vi "Lidar V4.0 RT Main.vi"() -> ()   [LabVIEW 2013]
uses:
  <vilib>/Platform/TimedLoop/XDataNode/timing_clust.ctl
  <vilib>/Platform/TimedLoop/XDataNode/nitl_modes.ctl
  <vilib>/Platform/TimedLoop/XDataNode/wakeup.ctl
  <vilib>/FPGAPlugInAG/PXIe-7962R/niLvFpga_Open_PXIe-7962R.vi
  <vilib>/rvi/interface/common/dynamic/niFpgaDynamicAddResources.vi
  <vilib>/FPGAPlugInAG/Dynamic/niLvFpga_Abort_Dynamic.vi
  <vilib>/FPGAPlugInAG/Dynamic/niLvFpga_Reset_Dynamic.vi
  <vilib>/rvi/interface/common/niFpgaWaitOnOcc.vi
  <vilib>/Utility/error.llb/Error Cluster From Error Code.vi
  <vilib>/FPGAPlugInAG/Dynamic/niLvFpga_Run_Dynamic.vi
  <vilib>/rvi/errors/niLvFpgaAdjustHostInterfaceError.vi
  <vilib>/Utility/file.llb/Read From Spreadsheet File (I64).vi
  <vilib>/FPGAPlugInAG/Dynamic/niLvFpga_Close_Dynamic.vi
  <vilib>/rvi/interface/nirviOpenFPGA/nirviOpenFPGA.xnode
  FPGA Bitfiles/GMLIDARV4_FPGATarget4_LIDARV4FPGAMain_YvCqZtg0Yfs.lvbitx
  FPGA/LIDAR V4 FPGA Main.vi
  <vilib>/rvi/interface/nirviMethod/nirviMethod.xnode
  <vilib>/Platform/TimedLoop/XDataNode/XDataNode.xnode
  <vilib>/rvi/interface/nirviReadWriteControl/nirviReadWriteControl.xnode
  <vilib>/rvi/interface/nirviCloseFPGA/nirviCloseFPGA.xnode
  <vilib>/rvi/errors/niLvFpgaMergeErrorWithErrorCode.vi
  NiFpgaLv.dll
  <vilib>/rvi/interface/Simulation/niFpgaSimulationCallBeginRW.vi
  <vilib>/Platform/TimedLoop/XDataNode/XDNodeRunTimeDep.lvlib
  <vilib>/FPGAPlugInAG/Dynamic/niLvFpga_StopFifo_Dynamic.vi
  <vilib>/FPGAPlugInAG/Dynamic/niLvFpga_ConfigureFifo_Dynamic.vi
  <vilib>/FPGAPlugInAG/Dynamic/niLvFpga_AcquireReadRegionFifo_Dynamic.vi
panel:
  in  "Read Scan File":bool
  out "Address":i16[](array[numeric])
  out "Array":i32[](array[numeric])
  out "x .and. y?":i32[][](graph)
  out "data":i16[](graph)
  in  "Read From Pattern File":bool
  out "Timeouts":u16
  out "Elements In Region":u32
  in  "Led Pattern":u8[](array[numeric])=[0, 44, 88, 132, 176, 220, 8, 52, 96, 140, 184, 228, 16, 60, 104, 148, 192, 236, 24, 68, 112, 156, 200, 244, 32, 76, 120, 164, 208, 252, 40, 84, 128, 172, 216, 4, 48, 92, 136, 180, 224, 12, 56, 100, 144, 188, 232, 20, 64, 108, 152, 196, 240, 28, 72, 116, 160, 204, 248, 36, 80, 124, 168, 212, 0, 44, 88, 132, 176, 220, 8, 52, 96, 140, 184, 228, 16, 60, 104, 148, 192, 236, 24, 68, 112, 156, 200, 244, 32, 76, 120, 164, 208, 252, 40, 84, 128, 172, 216, 4]
  in  "Fill Led Pattern":bool
  in  "# of Frames":u32=1 caption="# of Frames:"
  in  "Frames2File":bool
  in  "Fill VGA":bool
  in  "VGA data":i16[](array[numeric])=[0, 300, 600, 900, 1200, 1500, 1800, 2100, 2400, 2700, 3000, 3300, 3600, 3900, 4200, 4500, 4800, 5100, 5400, 5700, 6000, 6300, 6600, 6900, 7200, 7500, 7800, 8100, 8400, 8700, 9000, 9300, 9600, 9900, 10200, 10500, 10800, 11100, 11400, 11700, 12000, 12300, 12600, 12900, 13200, 13500, 13800, 14100, 14400, 14700, 15000, 15300, 15600, 15900, 16200, 16500, 16800, 17100, 17400, 17700, 18000, 18300, 18600, 18900, 19200, 19500, 19800, 20100, 20400, 20700, 21000, 21300, 21600, 21900, 22200, 22500, 22800, 23100, 23400, 23700, 24000, 24300, 24600, 24900, 25200, 25500, 25800, 26100, 26400, 26700, 27000, 27300, 27600, 27900, 28200, 28500, 28800, 29100, 29400, 29700]
  in  "PulsePerLed":i16=200 caption="Pulses Per Led"
  in  "ScanMode":bool
  in  "FrameStartDisable":bool=TRUE
  out "# of Frames 2":u32
  in  "Frames Stream":bool
  in  "Frames Period":i64=100
  out "Actual DMA Depth":u32=4000768
  out "Raw Data Timeouts":u16
  in  "StreamToRawFile":bool=TRUE
  out "Elements":i32=8192
  out "DiskWritesCounter":dbl=6240.0
  out "error out":errorcluster
  in  "Write To File":bool
  in  "Output file path":path=path "C:/Users/LIDAR/Desktop/Scans/Debug1.dat"
  out "Elements Remaining":u32
  in  "MaxStartSample":u8
  in  "ActiveLedIndex":u16=144
  in  "LedScanDebEn":bool
  in  "LaserPower 1":bool=TRUE
  in  "LaserPower 0":bool=TRUE
  in  "SampPerPattern":u32=4
  in  "stop":bool=TRUE
  # "Auto Actions"
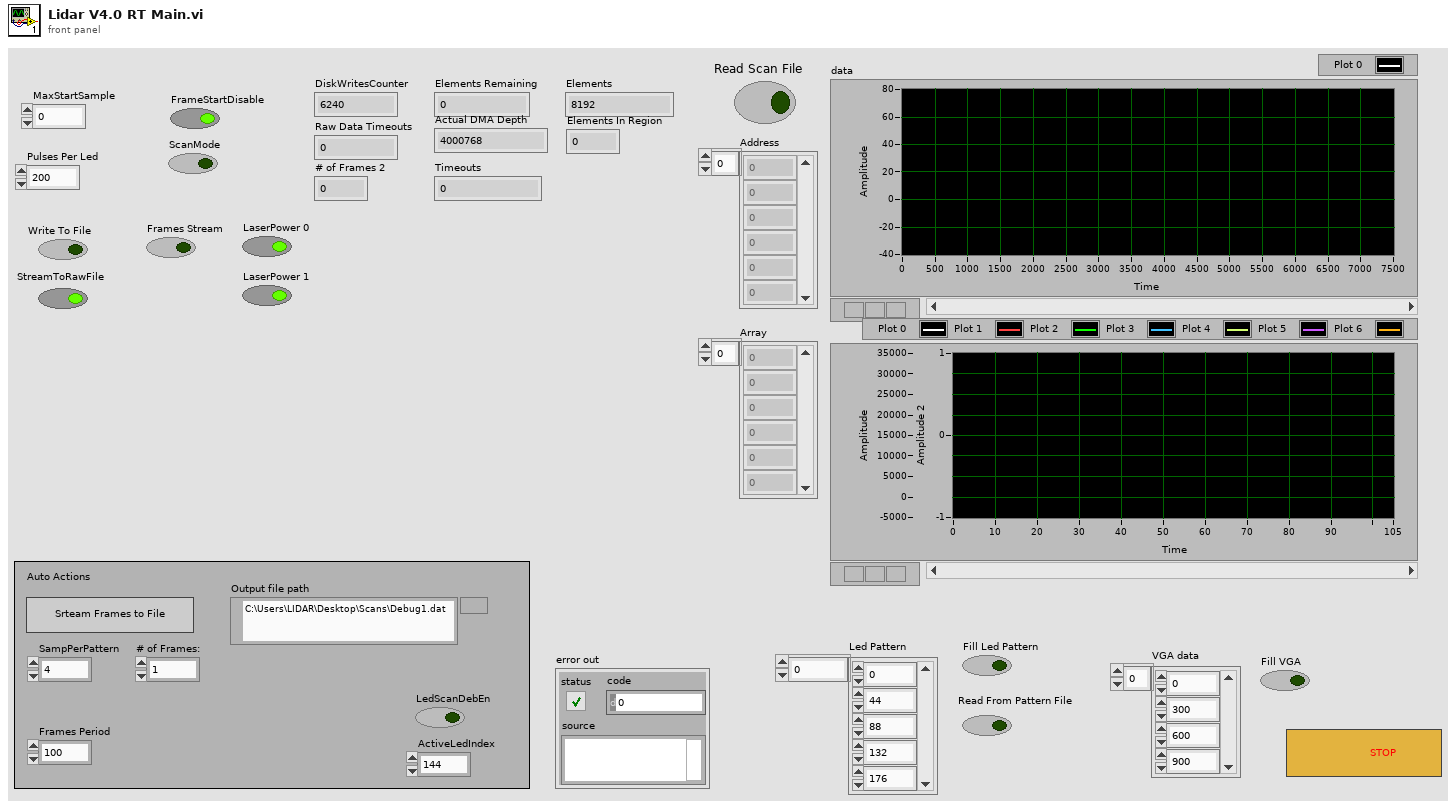
[diagram p1: front panel]
types:
  T1 = enum16{"open", "replace", "create", "open or create", "replace or create", "replace or create with confirmation"}
  T2 = typedef "XDNodeRunTimeDep.lvlib/timing_clust.ctl" = cluster{"Expected End [f-1]":u64, "Actual End [f-1]":u64, "Finished Late? [f-1]":bool, "Expected End [i-1]":u64, "Actual End [i-1]":u64, "Finished Late? [i-1]":bool, "Expected Start [i]":u64, "Actual Start [i]":u64, "Expected Start [f]":u64, "Actual Start [f]":u64, "Source Name":string, "Structure Name":string, "Period":i64, "Deadline":i64, "Offset":i64, "Start":i64, "Priority":i32, "Timeout":i32, "Mode":T3, "Wakeup Reason":T4, "Error":errorcluster, "Source Type":string, "Secondary Source Type":string, "Global End Time":u64, "Global Start Time":u64, "Frame Duration":u64, "Iteration Duration":u64, "Assigned CPU":i32, "I/O Scan Engine Mode":u32}
  T3 = typedef "XDNodeRunTimeDep.lvlib/nitl_modes.ctl" = enum32{"No Change", "Process missed periods, maintain original phase", "Discard missed periods, maintain original phase", "Process missed periods, ignore original phase", "Discard missed periods, ignore original phase"}
  T4 = typedef "XDNodeRunTimeDep.lvlib/wakeup.ctl" = enum32{"Normal", "Aborted", "Asynchronous wakeup", "Timing source error", "Timed loop error", "Timeout"}
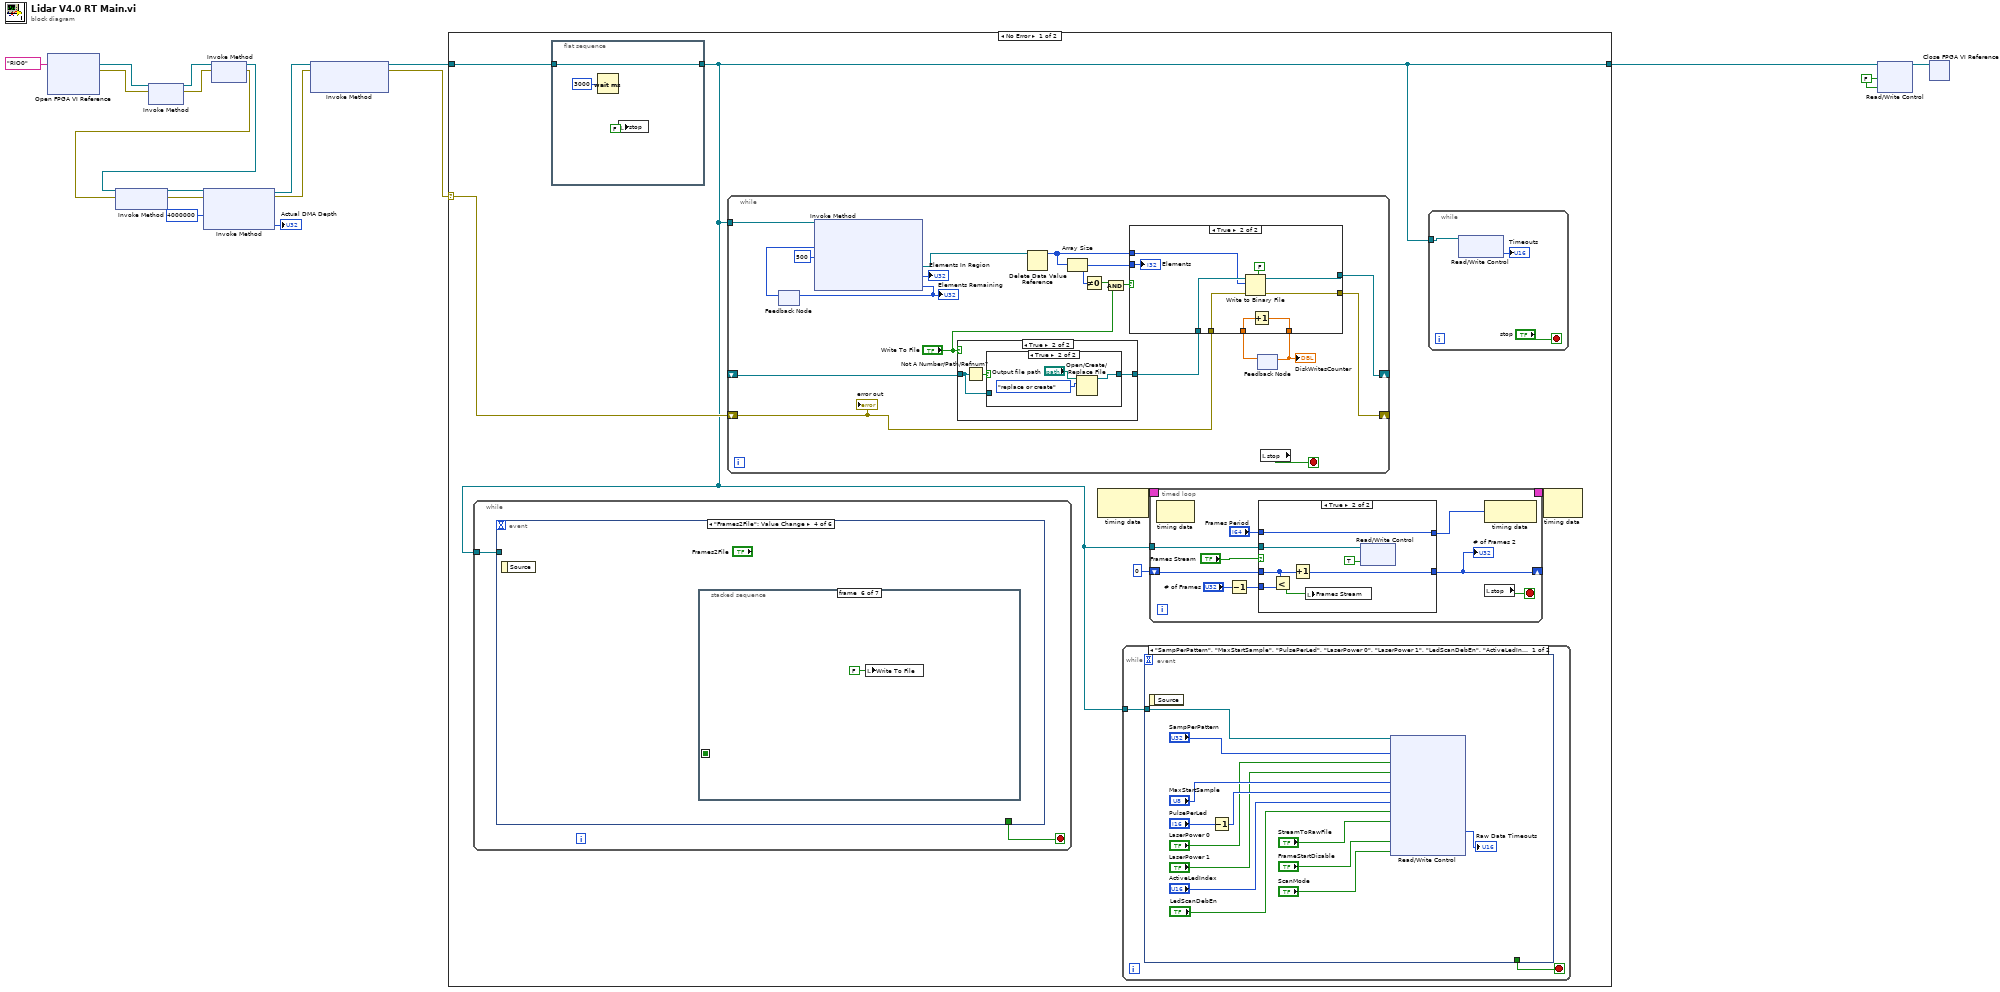
[diagram p0: block diagram]
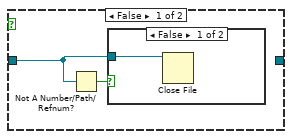
[diagram p2: hidden frame]
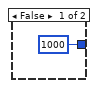
[diagram p6: hidden frame]
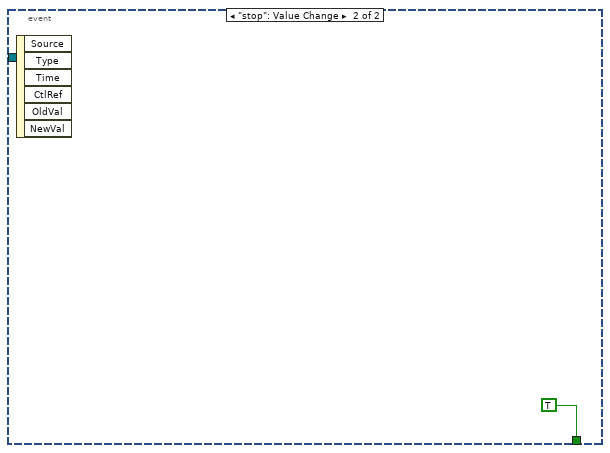
[diagram p7: hidden frame]
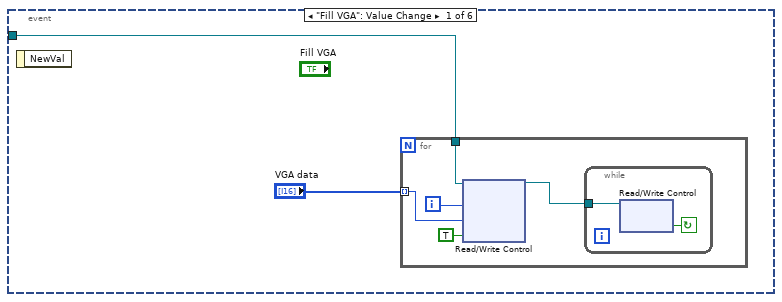
[diagram p8: hidden frame]
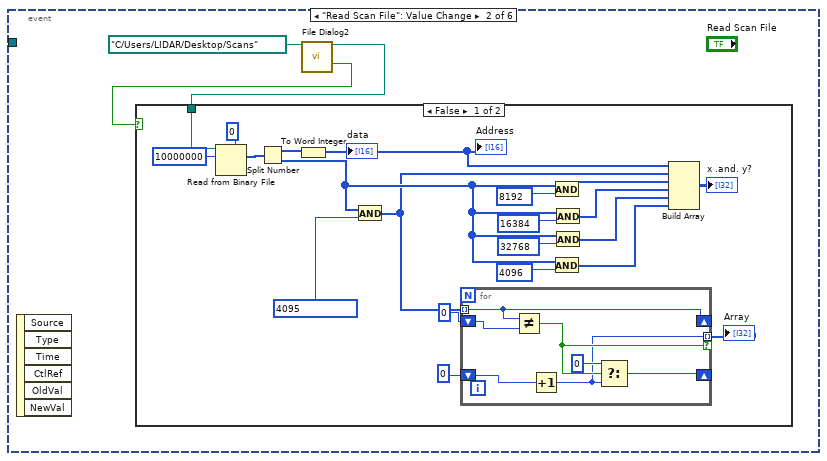
[diagram p9: hidden frame]
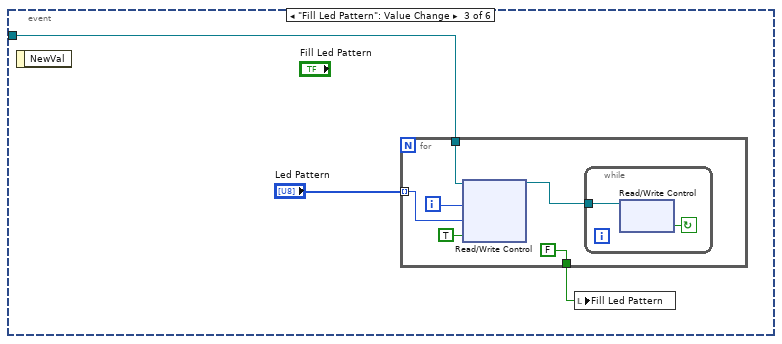
[diagram p11: hidden frame]
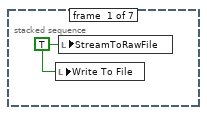
[diagram p12: hidden frame]
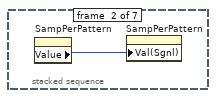
[diagram p13: hidden frame]
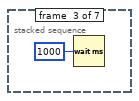
[diagram p14: hidden frame]
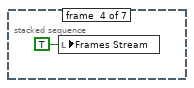
[diagram p15: hidden frame]
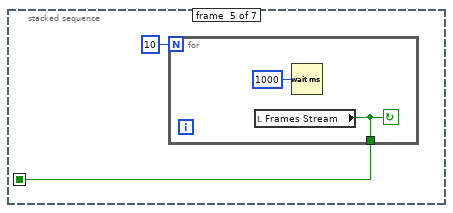
[diagram p16: hidden frame]
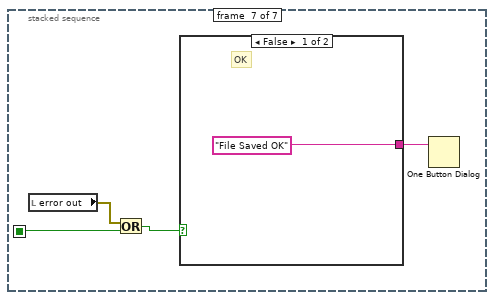
[diagram p17: hidden frame]
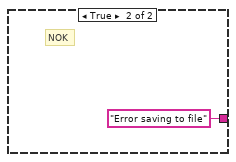
[diagram p18: hidden frame]
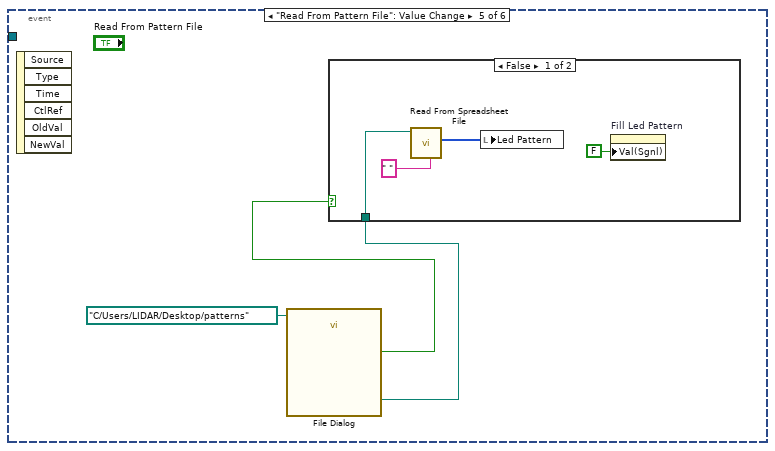
[diagram p19: hidden frame]
diagram:
  w8 = FALSE ("PFI2")
  n1 = xnode "Open FPGA VI Reference"("resource name"=tag "RIO0") -> ("FPGA VI Reference Out"=w16:refnum<k20>, "error out"=w14:errorcluster)  [unwired: 1 in]
  n2 = xnode "Invoke Method"("FPGA VI Reference In"=w16, "error in"=w14) -> ("FPGA VI Reference Out"=w15:refnum<k20>, "error out"=w13:errorcluster)
  n3 = xnode "Invoke Method"("FPGA VI Reference In"=w15, "error in"=w13) -> ("FPGA VI Reference Out"=w6:refnum<k20>, "error out"=w5:errorcluster)
  n4 = xnode "Invoke Method"("FPGA VI Reference In"=w6, "error in"=w5) -> ("FPGA VI Reference Out"=w11:refnum<k20>, "error out"=w12:errorcluster)
  n5 = xnode "Invoke Method"("FPGA VI Reference In"=w11, "error in"=w12, "Requested Depth"=u32 4000000) -> ("FPGA VI Reference Out"=w2:refnum<k20>, "error out"=w1:errorcluster, "Actual Depth"=→"Actual DMA Depth":u32)
  n6 = xnode "Invoke Method"("FPGA VI Reference In"=w2, "error in"=w1) -> ("FPGA VI Reference Out"=w4:refnum<k20>, "error out"=w3:errorcluster)  [unwired: 1 in]
  n7 = case shown="No Error" w3 {
    selector: w3 -> [w23 w187]
    tunnel: [w19 w188] -> w17
    tunnel: w4 -> [w24 w188]
    frame No Error {
      n8 = while {
        tunnel: w19 -> [w109]
        stop <- w108 stop-if-true
        n9 = event shown="[3] \"Frames2File\": Value Change" {
          selector: _ -> [_ _ _ _ _ _]
          dyn-events: _ -> [_ _ _ _ _ _]
          timeout: _ -> [_ _ _ _ _ _]
          tunnel: w109 -> [w110 _ w151 _ _ _]
          tunnel: [_ _ _ _ _ TRUE] -> w108
          event "Fill VGA": Value Change {
            n10 = event-data() -> ()  [unwired: 1 in, 1 out]
            n11 = for {
              tunnel: w110 -> [w116]
              tunnel: "VGA data" -> [w115] mode=indexing
              i -> [w114]
              n12 = xnode "Read/Write Control"("FPGA VI Reference In"=w116, "VgaAdd"=w114, "VgaData"=w115, "FillVga"=TRUE) -> ("FPGA VI Reference Out"=w113:refnum<k20>)  [unwired: 1 in, 1 out]
              n13 = while {
                tunnel: w113 -> [w118]
                stop <- w117 continue-if-true
                n14 = xnode "Read/Write Control"("FPGA VI Reference In"=w118) -> ("FillVga"=w117:bool)  [unwired: 1 in, 2 out]
              }
            }
          }
          event "Read Scan File": Value Change {
            n15 = event-data() -> ()  [unwired: 1 in, 6 out]
            n16 = call "File Dialog2"("start path"=path "C:/Users/LIDAR/Desktop/Scans") -> ("selected path"=w119:path, "cancelled"=w120:bool)  [unwired: 11 in, 2 out]
            n17 = case shown="False" w120 {
              tunnel: w119 -> [w122 _]
              frame False {
                n18 = Read from Binary File(5:u32 0, 10:10000000 ("count (1)"), 11:w122) -> (2:w125:u32[])  [unwired: 3 in, 3 out]
                n19 = Split Number(x=w125) -> (hi(x)=w126:u16[], lo(x)=w141:u16[])
                n20 = To Word Integer(number=w126) -> (16bit integer=w132:i16[])
                "data" <- w132
                "Address" <- w132
                n21 = And(x=w141, y=4095) -> (x .and. y?=w130:i32[])
                n22 = for {
                  tunnel: w130 -> [w149] mode=indexing
                  shift-right: [w149] -> _
                  shift-left: 0 -> [w148]
                  shift-right: [w144] -> _
                  shift-left: 0 -> [w147]
                  tunnel: [w143] -> w131 mode=indexing if=w145
                  n23 = Not Equal?(x=w149, y=w148) -> (x != y?=w145:bool)
                  n24 = Increment(x=w147) -> (x+1=w143:i32)
                  n25 = Select(t=0, s=w145, f=w143) -> (s? t:f=w144:i32)
                }
                "Array" <- w131
                n26 = And(x=w141, y=8192) -> (x .and. y?=w136:i32[])
                n27 = And(x=w141, y=4096) -> (x .and. y?=w142:i32[])
                n28 = And(x=w141, y=16384) -> (x .and. y?=w137:i32[])
                n29 = And(x=w141, y=32768) -> (x .and. y?=w139:i32[])
                n30 = Build Array(w132, w130, w136, w137, w139, w142) -> (→"x .and. y?":i32[][])
              }
              frame True {
              }
            }
          }
          event "Fill Led Pattern": Value Change {
            n31 = event-data() -> ()  [unwired: 1 in, 1 out]
            n32 = for {
              tunnel: w151 -> [w158]
              tunnel: "Led Pattern" -> [w157] mode=indexing
              tunnel: [FALSE ("Fill Led Pattern")] -> w150
              i -> [w156]
              n33 = xnode "Read/Write Control"("FPGA VI Reference In"=w158, "PattAdd"=w156, "PattData"=w157, "FillPatt"=TRUE ("FillVga")) -> ("FPGA VI Reference Out"=w155:refnum<k20>)  [unwired: 1 in, 1 out]
              n34 = while {
                tunnel: w155 -> [w160]
                stop <- w159 continue-if-true
                n35 = xnode "Read/Write Control"("FPGA VI Reference In"=w160) -> ("FillPatt"=w159:bool)  [unwired: 1 in, 2 out]
              }
            }
            n36 = local write "Fill Led Pattern"(w150) -> ()
          }
          event "Frames2File": Value Change {
            n37 = event-data() -> ()  [unwired: 1 in, 1 out]
            n38 = stacked-sequence {
              seq-local: [_ _ _ _ w165 _ _] -> [_ _ _ _ _ _ w173]
              frame #0 {
                w161 = TRUE ("StreamToRawFile")
                n39 = local write "Write To File"(w161) -> ()
                n40 = local write "StreamToRawFile"(w161) -> ()
              }
              frame #1 {
                n41 = property on="SampPerPattern" class="DigNum (strict)"() -> ("Value"=w162:u32)  [unwired: 2 in, 2 out]
                n42 = property on="SampPerPattern" class="DigNum (strict)"("Val(Sgnl)"=w162) -> ()  [unwired: 2 in, 2 out]
              }
              frame #2 {
                n43 = Wait (ms)(milliseconds to wait=u32 1000) -> ()  [unwired: 1 out]
              }
              frame #3 {
                n44 = local write "Frames Stream"(TRUE ("Frames Stream")) -> ()
              }
              frame #4 {
                n45 = for {
                  N: 10 -> [_]
                  tunnel: [w167] -> w165
                  stop <- w167 continue-if-true
                  n46 = local read "Frames Stream"() -> (w167:bool)
                  n47 = Wait (ms)(milliseconds to wait=u32 1000) -> ()  [unwired: 1 out]
                }
              }
              frame #5 {
                n48 = local write "Write To File"(FALSE ("Write To File")) -> ()
              }
              frame #6 {
                n49 = local read "error out"() -> (w170:errorcluster)
                n50 = Or(x=w170, y=w173) -> (x .or. y?=w171:bool)
                n51 = case shown="False" w171 {
                  tunnel: ["File Saved OK" ("message") "Error saving to file" ("message")] -> w172
                  frame False {
                    # "OK"
                  }
                  frame True {
                    # "NOK"
                  }
                }
                n52 = One Button Dialog(message=w172) -> ()  [unwired: 1 in, 1 out]
              }
            }
          }
          event "Read From Pattern File": Value Change {
            n53 = event-data() -> ()  [unwired: 1 in, 6 out]
            n54 = call "File Dialog"("start path"=path "C:/Users/LIDAR/Desktop/patterns") -> ("selected path"=w176:path, "cancelled"=w177:bool)  [unwired: 11 in, 2 out]
            n55 = case shown="False" w177 {
              tunnel: w176 -> [w179 _]
              frame False {
                n56 = call-poly <vilib>:"Read From Spreadsheet File.vi"("delimiter (\\t)"=" " ("delimiter (\\t)"), "file path (dialog if empty)"=w179) -> ("first row"=w182:i64[])  [unwired: 5 in, 4 out]
                n57 = local write "Led Pattern"(w182) -> ()
                n58 = property on="Fill Led Pattern" class="Bool (strict)"("Val(Sgnl)"=FALSE ("Value (Signaling)")) -> ()  [unwired: 2 in, 2 out]
              }
              frame True {
              }
            }
          }
          event "stop": Value Change {
            n59 = event-data() -> ()  [unwired: 1 in, 6 out]
          }
        }
      }
      n60 = flat-sequence {
        tunnel: [w186] -> w19
        tunnel: w24 -> [w186]
        frame #0 {
          n61 = Wait (ms)(milliseconds to wait=u32 3000) -> ()  [unwired: 1 out]
          n62 = local write "stop"(FALSE ("stop")) -> ()
        }
      }
      n63 = while {
        tunnel: w19 -> [w25]
        shift-right: [w43] -> _
        shift-left: _ -> [w36]
        shift-right: [w42] -> _
        shift-left: w23 -> [w41]
        stop <- w31 stop-if-true
        n64 = feedback #1() -> (w29:u32)  [unwired: 1 in]
        n65 = xnode "Invoke Method"("FPGA VI Reference In"=w25, "Number of Elements"=w29, "Timeout (ms)"=500) -> ("Read Region Reference"=w38:refnum<data-value>, "Elements In Region"=→"Elements In Region":u32, "Elements Remaining"=w26:u32)  [unwired: 1 in, 2 out]
        "Elements Remaining" <- w26
        n66 = feedback-in #1(w26) -> ()
        n67 = case shown="True" "Write To File" {
          tunnel: w36 -> [w44 w47]
          tunnel: [_ w49] -> w35
          frame False {
            n68 = Not A Number/Path/Refnum?(number/path/refnum=w44) -> (NaN/Path/Refnum?=w45:bool)
            n69 = case shown="False" w45 {
              tunnel: w44 -> [w46 _]
              frame False {
                n70 = Close File(refnum=w46) -> ()  [unwired: 1 in, 2 out]
              }
              frame True {
              }
            }
          }
          frame True {
            n71 = Not A Number/Path/Refnum?(number/path/refnum=w47) -> (NaN/Path/Refnum?=w48:bool)
            n72 = case shown="True" w48 {
              tunnel: [w50 w51] -> w49
              tunnel: w47 -> [w50 _]
              frame False {
              }
              frame True {
                n73 = Open/Create/Replace File(file path (use dialog)="Output file path", operation (0:open)=T1."replace or create") -> (refnum out=w51:refnum<file>)  [unwired: 4 in, 2 out]
              }
            }
          }
        }
        n74 = Delete Data Value Reference(data value reference=w38) -> (data value=w34:u32[])  [unwired: 1 in, 1 out]
        n75 = Array Size(array=w34) -> (size(s)=w33:i32)
        n76 = Not Equal To 0?(x=w33) -> (x != 0?=w32:bool)
        n77 = And(x=w32, y="Write To File") -> (x .and. y?=w37:bool)
        n78 = feedback #2() -> (w39:dbl)  [unwired: 1 in]
        n79 = case shown="True" w37 {
          tunnel: [w54 w64] -> w43
          tunnel: w41 -> [w56 w59]
          tunnel: [w56 w63] -> w42
          tunnel: [w55 w61] -> w40
          tunnel: w39 -> [w55 w62]
          tunnel: w34 -> [_ w58]
          tunnel: w35 -> [w54 w60]
          tunnel: w33 -> [_ w57]
          frame False {
          }
          frame True {
            n80 = Write to Binary File(file (use dialog)=w60, data=w58, error in=w59, 5:FALSE ("prepend array or string size? (T)")) -> (refnum out=w64:refnum<file>, error out=w63:errorcluster)  [unwired: 2 in, 1 out]
            n81 = Increment(x=w62) -> (x+1=w61:dbl)
            "Elements" <- w57
          }
        }
        "DiskWritesCounter" <- w40
        n82 = feedback-in #2(w40) -> ()
        n83 = local read "stop"() -> (w31:bool)
        "error out" <- w41
      }
      n84 = node-c288() -> (w22:T2)  [unwired: 1 in]
      n85 = while {
        tunnel: w19 -> [w92]
        stop <- w93 stop-if-true
        n86 = event shown="[0] \"SampPerPattern\", \"MaxStartSample\", \"PulsePerLed\", \"LaserPower 0\", \"LaserPower 1\", \"LedScanDebEn\", \"ActiveLedIndex\", \"StreamToRawFile\", \"FrameStartDisable\", \"ScanMode\": Value Change" {
          selector: _ -> [_ _]
          dyn-events: _ -> [_ _]
          timeout: _ -> [_ _]
          tunnel: [_ TRUE] -> w93
          tunnel: w92 -> [w97 _]
          event "SampPerPattern", "MaxStartSample", "PulsePerLed", "LaserPower 0", "LaserPower 1", "LedScanDebEn", "ActiveLedIndex", "StreamToRawFile", "FrameStartDisable", "ScanMode": Value Change {
            n87 = event-data() -> ()  [unwired: 1 in, 1 out]
            n88 = Decrement(x="PulsePerLed") -> (x-1=w106:i16)
            n89 = xnode "Read/Write Control"("FPGA VI Reference In"=w97, "SampPerPattern"="SampPerPattern", "PFI2"="LaserPower 0", "PFI3"="LaserPower 1", "MaxStartSample"="MaxStartSample", "PulsePerLed"=w106, "ActiveLedIndex"="ActiveLedIndex", "LedScanDebEn"="LedScanDebEn", "StreamToDMA"="StreamToRawFile", "FrameStartDisable"="FrameStartDisable", "ScanMode"="ScanMode") -> ("Timeouts"=→"Raw Data Timeouts":u16)  [unwired: 1 in, 2 out]
          }
          event "stop": Value Change {
            n90 = event-data() -> ()  [unwired: 1 in, 6 out]
          }
        }
      }
      n91 = timed-loop {
        timing: w22 -> [_]
        timing-out: [_] -> w21
        tunnel: w19 -> [w77]
        shift-right: [w72] -> _
        shift-left: u32 0 ("# of Frames") -> [w73]
        stop <- w74 stop-if-true
        n92 = node-c288() -> ()  [unwired: 1 in, 1 out]
        n93 = Decrement(x="# of Frames") -> (x-1=w69:u32)
        n94 = case shown="True" "Frames Stream" {
          tunnel: w77 -> [_ w85]
          tunnel: [i64 1000 ("Frames Period") w84] -> w75
          tunnel: "Frames Period" -> [_ w84]
          tunnel: w73 -> [_ w80]
          tunnel: [_ w83] -> w72
          tunnel: w69 -> [_ w81]
          frame False {
          }
          frame True {
            n95 = Less?(x=w80, y=w81) -> (x < y?=w79:bool)
            n96 = Increment(x=w80) -> (x+1=w83:u32)
            n97 = local write "Frames Stream"(w79) -> ()
            n98 = xnode "Read/Write Control"("FPGA VI Reference In"=w85, "Start"=TRUE ("SingleFrame")) -> ()  [unwired: 1 in, 2 out]
          }
        }
        "# of Frames 2" <- w72
        n99 = node-c288(w75) -> ()  [unwired: 1 out]
        n100 = local read "stop"() -> (w74:bool)
      }
      n101 = while {
        tunnel: w19 -> [w68]
        stop <- "stop" stop-if-true
        n102 = xnode "Read/Write Control"("FPGA VI Reference In"=w68) -> ("Timeouts"=→"Timeouts":u16)  [unwired: 1 in, 2 out]
      }
      n103 = node-c288(w21) -> ()  [unwired: 1 out]
    }
    frame Error {
      n104 = local write "error out"(w187) -> ()
    }
  }
  n105 = xnode "Read/Write Control"("FPGA VI Reference In"=w17, "PFI2"=w8, "PFI3"=w8) -> ("FPGA VI Reference Out"=w7:refnum<k20>)  [unwired: 1 in, 1 out]
  n106 = xnode "Close FPGA VI Reference"("FPGA VI Reference In"=w7) -> ()  [unwired: 1 in, 1 out]
